vi "Format File Property.vi"(8 "Error In":errorcluster, 9 "File Property Value":string, 10 "File Property Name":string, 11 "String in":string) -> (0 "Error Out":errorcluster, 3 "String out":string)   [LabVIEW 2018]
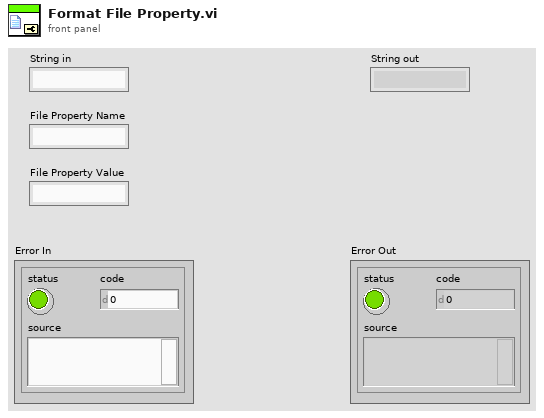
[diagram p1: front panel]
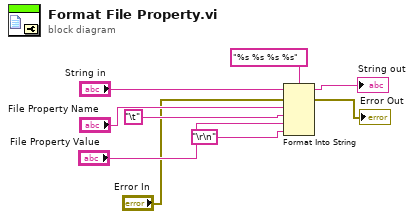
[diagram p0: block diagram]
diagram:
  n1 = Format Into String(format string="%s %s %s %s", initial string="String in", error in="Error In", "File Property Name", "\t", "File Property Value", "\r\n") -> (resulting string=→"String out":string, error out=→"Error Out":errorcluster)
